vi "Completed.vi"(8 "error in (no error)":errorcluster, 11 "MovementInstruction.lvclass 2":refnum<class "MovementInstruction.lvclass">) -> (0 "error out":errorcluster, 3 "Completed":bool)   [LabVIEW 2015, in "MovementInstruction.lvclass"]
uses:
  MovementInstruction.lvclass
  MovementInstruction.lvclass/MovementInstruction.ctl
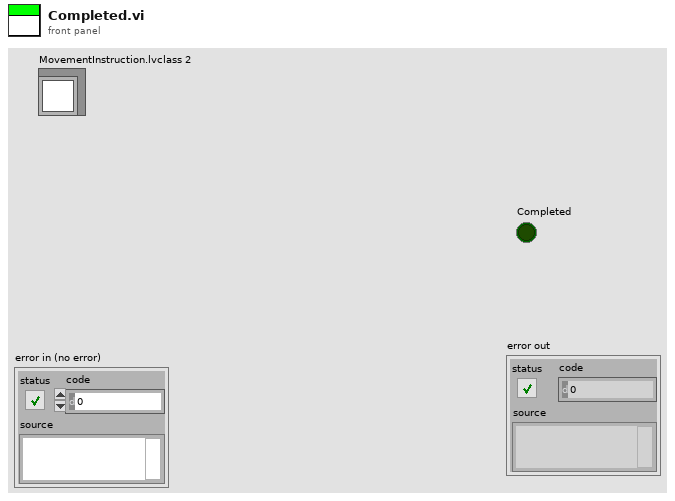
[diagram p1: front panel]
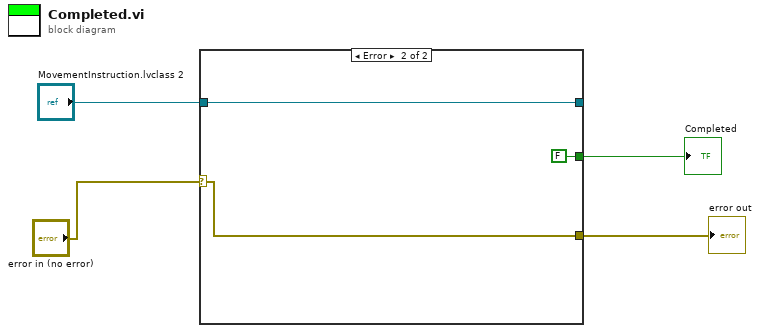
[diagram p0: block diagram]
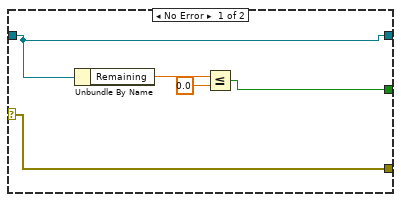
[diagram p2: hidden frame]
diagram:
  n1 = case shown="Error" "error in (no error)" {
    selector: "error in (no error)" -> [w9 w11]
    tunnel: [w8 w12] -> _
    tunnel: "MovementInstruction.lvclass 2" -> [w8 w12]
    tunnel: [w9 w11] -> w2
    tunnel: [w5 FALSE] -> w1
    frame No Error {
      n2 = Unbundle By Name(w8) -> ("Remaining"=w7:dbl)
      n3 = Less Or Equal?(x=w7, y=0.0) -> (x <= y?=w5:bool)
    }
    frame Error {
    }
  }
  "error out" <- w2
  "Completed" <- w1
